vi "transmitSceneWithRetry.vi"(10 "scene #":i32, 11 "24-bit pixmap":u32[][](array[numeric])) -> (0 "error out":errorcluster)   [LabVIEW 2014]
uses:
  typeDefs/pixxelAction.ctl
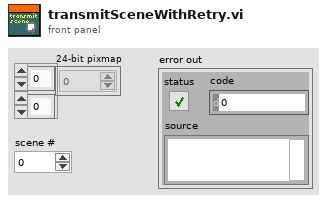
[diagram p1: front panel]
types:
  T1 = typedef "pixxelAction.ctl" = enum16{"init", "watchdog", "headScene", "setPixel", "tailScene", "headProg", "tailProg", "showSceneFrame", "black", "playFrames", "close", "uploadProg", "startProg", "pauseProg", "stopProg", "jumpTo", "setIP", "setGW", "initFlash", "saveScene", "saveProgram"}
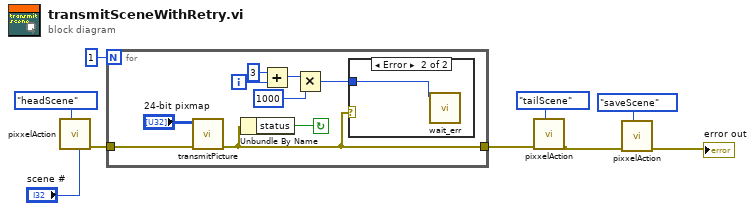
[diagram p0: block diagram]
diagram:
  n1 = call "pixxelAction.vi"("u16"="scene #", "PIXXELaction"=pixxelAction."headScene") -> ("error out"=w7:errorcluster)  [unwired: 9 in]
  n2 = for {
    N: 1 -> [_]
    tunnel: [w16] -> w4
    tunnel: w7 -> [w10]
    i -> [w15]
    stop <- w17 continue-if-true
    n3 = call "transmitPicture.vi"("error in (no error)"=w10, "24-bit pixmap"="24-bit pixmap") -> ("error out"=w16:errorcluster)  [unwired: 9 in]
    n4 = Unbundle By Name(w16) -> ("status"=w17:bool)
    n5 = Add(x=3, y=w15) -> (x+y=w14:i32)
    n6 = Multiply(x=w14, y=1000) -> (x*y=w12:i32)
    n7 = case shown="Error" w16 {
      tunnel: w12 -> [_ w19]
      frame No Error {
      }
      frame Error {
        n8 = call <userlib>:"wait_err.vi"("milliseconds to wait"=w19) -> ()  [unwired: 10 in, 1 out]
      }
    }
  }
  n9 = call "pixxelAction.vi"("PIXXELaction"=pixxelAction."tailScene", "error in (no error)"=w4) -> ("error out"=w2:errorcluster)  [unwired: 9 in]
  n10 = call "pixxelAction.vi"("PIXXELaction"=pixxelAction."saveScene", "error in (no error)"=w2) -> ("error out"=→"error out":errorcluster)  [unwired: 9 in]
